vi "TelemetryServer_MultiplexerStop.vi"(3 "Multiplexer":T1, 9 "Error out":errorcluster caption="error in (no error)") -> (6 "error out":errorcluster)   [LabVIEW 2009]
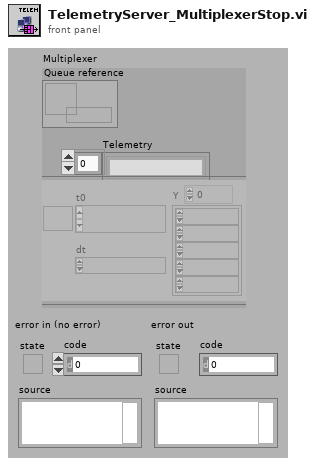
[diagram p1: front panel]
types:
  T1 = cluster{"Queue reference":refnum<queue>, "Telemetry":string[], "Queuers references":refnum<vi>[], "Waveforms":waveform(dbl)[]}
  T2 = enum32{"Bad", "Idle", "Run top level", "Running"}
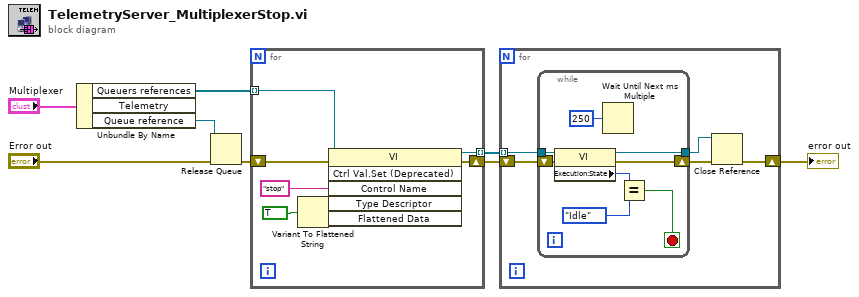
[diagram p0: block diagram]
diagram:
  n1 = Unbundle By Name("Multiplexer") -> ("Queuers references"=w1:refnum<vi>[], "Queue reference"=w2:refnum<queue>)  [unwired: 1 out]
  n2 = Release Queue(queue=w2, error in (no error)="Error out") -> (error out=w3:errorcluster)  [unwired: 3 out]
  n3 = for {
    tunnel: [w16] -> w8 mode=indexing
    shift-right: [w15] -> w7
    shift-left: w3 -> [w9]
    tunnel: w1 -> [w10] mode=indexing
    n4 = Variant To Flattened String(Variant=TRUE) -> (data string=w13:string, 1:w12:i16[])
    n5 = invoke class="VI" method="Ctrl Val.Set (Deprecated)"(reference=w10, error in=w9, "Control Name"="stop" ("Nom de la commande"), "Type Descriptor"=w12, "Flattened Data"=w13) -> (reference out=w16:refnum<vi>, error out=w15:errorcluster)  [unwired: 1 in, 4 out]
  }
  n6 = for {
    tunnel: w8 -> [w19] mode=indexing
    shift-right: [w17] -> w6
    shift-left: w7 -> [w18]
    n7 = while {
      tunnel: w19 -> [w28]
      tunnel: [w23] -> w21
      shift-right: [w22] -> w20
      shift-left: w18 -> [w29]
      stop <- w24 stop-if-true
      n8 = property class="VI"(reference=w28, error in=w29) -> (reference out=w23:refnum<vi>, error out=w22:errorcluster, "Execution:State"=w27:T2)
      n9 = Wait Until Next ms Multiple(millisecond multiple=u32 250 ("n millisecondes")) -> ()  [unwired: 1 out]
      n10 = Equal?(x=w27, y=T2."Idle" ("Exécution : état")) -> (x = y?=w24:bool)
    }
    n11 = Close Reference(reference=w21, error in (no error)=w20) -> (error out=w17:errorcluster)
  }
  "error out" <- w6
